vi "Matrix_display_target.vi"() -> ()   [LabVIEW 2013]
uses:
  <vilib>/Platform/TimedLoop/XDataNode/timing_clust.ctl
  <vilib>/Platform/TimedLoop/XDataNode/nitl_modes.ctl
  <vilib>/Platform/TimedLoop/XDataNode/wakeup.ctl
  <vilib>/rvi/Emulation/niFpgaSctlEmulationGetInTimedLoop.vi
  <vilib>/rvi/Emulation/niFpgaProcessEmulError.vi
  <vilib>/rvi/Emulation/niFpgaEmulationReportErrorSimple.vi
  <vilib>/rvi/Emulation/niFpgaGetClockAttributes.vi
  <vilib>/rvi/Emulation/niFpgaCriticalErrorInLSC.vi
  <vilib>/rvi/eio/common/nirviEmuTemplateMethod_errors.vi
  <vilib>/rvi/interface/RandomDataEmulation/nirviRandomDataFPGAFIFO.vi
  <vilib>/rvi/interface/RandomDataEmulation/niFpgaRandomDataHandleErrors.vi
  <vilib>/Platform/TimedLoop/XDataNode/XDataNode.xnode
  <vilib>/eio/EIONode/EIONode.xnode
  <vilib>/rvi/DataTransferAndStorage/Container/XNode/niFpgaContainer.xnode
  <vilib>/rvi/interface/RandomDataEmulation/nirviRandomDataFpgaReadWriteTemplate.vi
  <vilib>/Platform/TimedLoop/XDataNode/XDNodeRunTimeDep.lvlib
panel:
  out "String_counter":i16
  in  "String_number":i16
  in  "I2C_Write":bool
  in  "Read2":u8 format="%x"
  in  "Read1":u8 format="%x"
  in  "Device_Read":u8=187 format="%x"
  in  "Reg":u8=9 format="%x"
  in  "Device_Write":u8=186 format="%x"
  in  "89":i16=89
  in  "100_Sclk_divider":i32=25
  out "Sclk":bool
  in  "75_Stop":i16=75
  in  "53":i16=53
  in  "35":i16=35
  in  "17":i16=17
  in  "71":i16=71
  in  "54":i16=54
  in  "36":i16=36
  in  "18":i16=18
  in  "72":i16=72
  in  "50_Rise/Fall divider":i32=50
  in  "0_WE divider":i32
  in  "DataUp":u64
  in  "DataLow":u64
  out "ACK":bool[](array[boolean])
  out "Data_Array":bool[](array[boolean])
  in  "I2C_Request":bool
  in  "FALSE_LV":bool
  in  "FALSE_PIXCLK":bool
  in  "TRUE_FV":bool
  in  "Линия_ прочтена":bool
  in  "Остановите":bool
  out "Линия_готова_на_все":bool
  in  "Читай_Линию":bool
  in  "1_EXTCLK_divider":i16=2
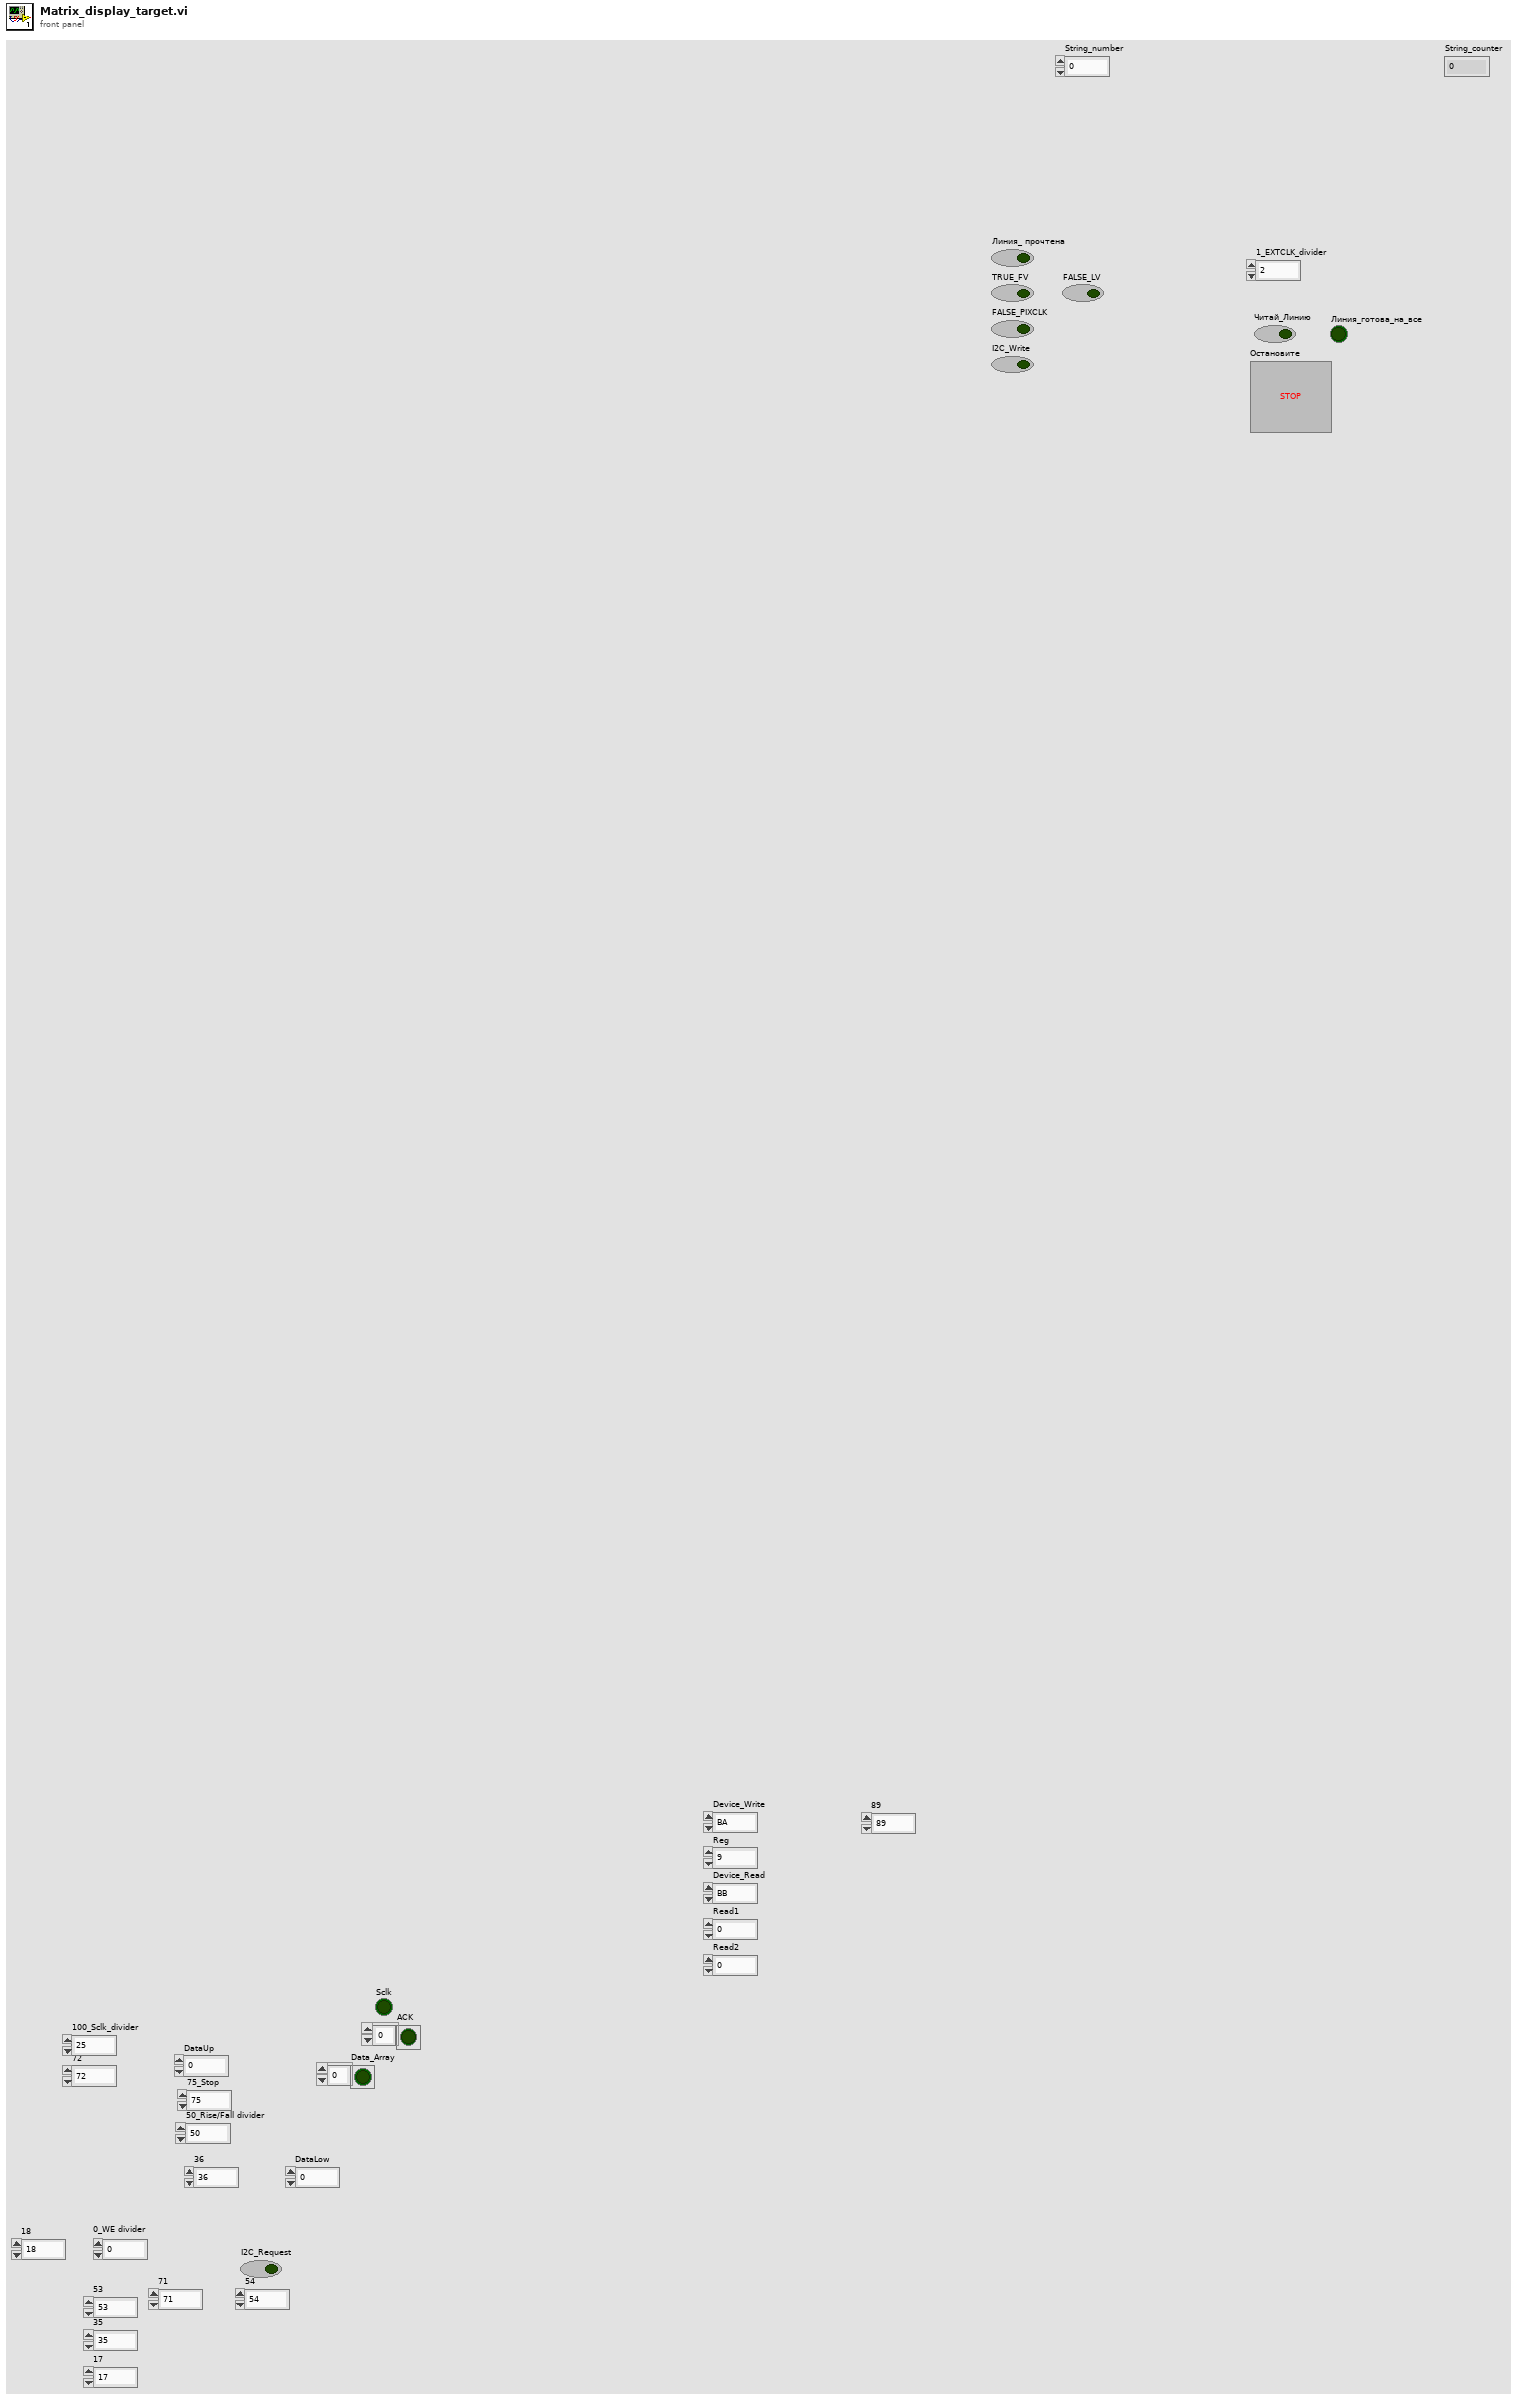
[diagram p1: front panel]
types:
  T1 = typedef "XDNodeRunTimeDep.lvlib/timing_clust.ctl" = cluster{"Expected End [f-1]":u64, "Actual End [f-1]":u64, "Finished Late? [f-1]":bool, "Expected End [i-1]":u64, "Actual End [i-1]":u64, "Finished Late? [i-1]":bool, "Expected Start [i]":u64, "Actual Start [i]":u64, "Expected Start [f]":u64, "Actual Start [f]":u64, "Source Name":string, "Structure Name":string, "Period":i64, "Deadline":i64, "Offset":i64, "Start":i64, "Priority":i32, "Timeout":i32, "Mode":T2, "Wakeup Reason":T3, "Error":errorcluster, "Source Type":string, "Secondary Source Type":string, "Global End Time":u64, "Global Start Time":u64, "Frame Duration":u64, "Iteration Duration":u64, "Assigned CPU":i32, "I/O Scan Engine Mode":u32}
  T2 = typedef "XDNodeRunTimeDep.lvlib/nitl_modes.ctl" = enum32{"No Change", "Process missed periods, maintain original phase", "Discard missed periods, maintain original phase", "Process missed periods, ignore original phase", "Discard missed periods, ignore original phase"}
  T3 = typedef "XDNodeRunTimeDep.lvlib/wakeup.ctl" = enum32{"Normal", "Aborted", "Asynchronous wakeup", "Timing source error", "Timed loop error", "Timeout"}
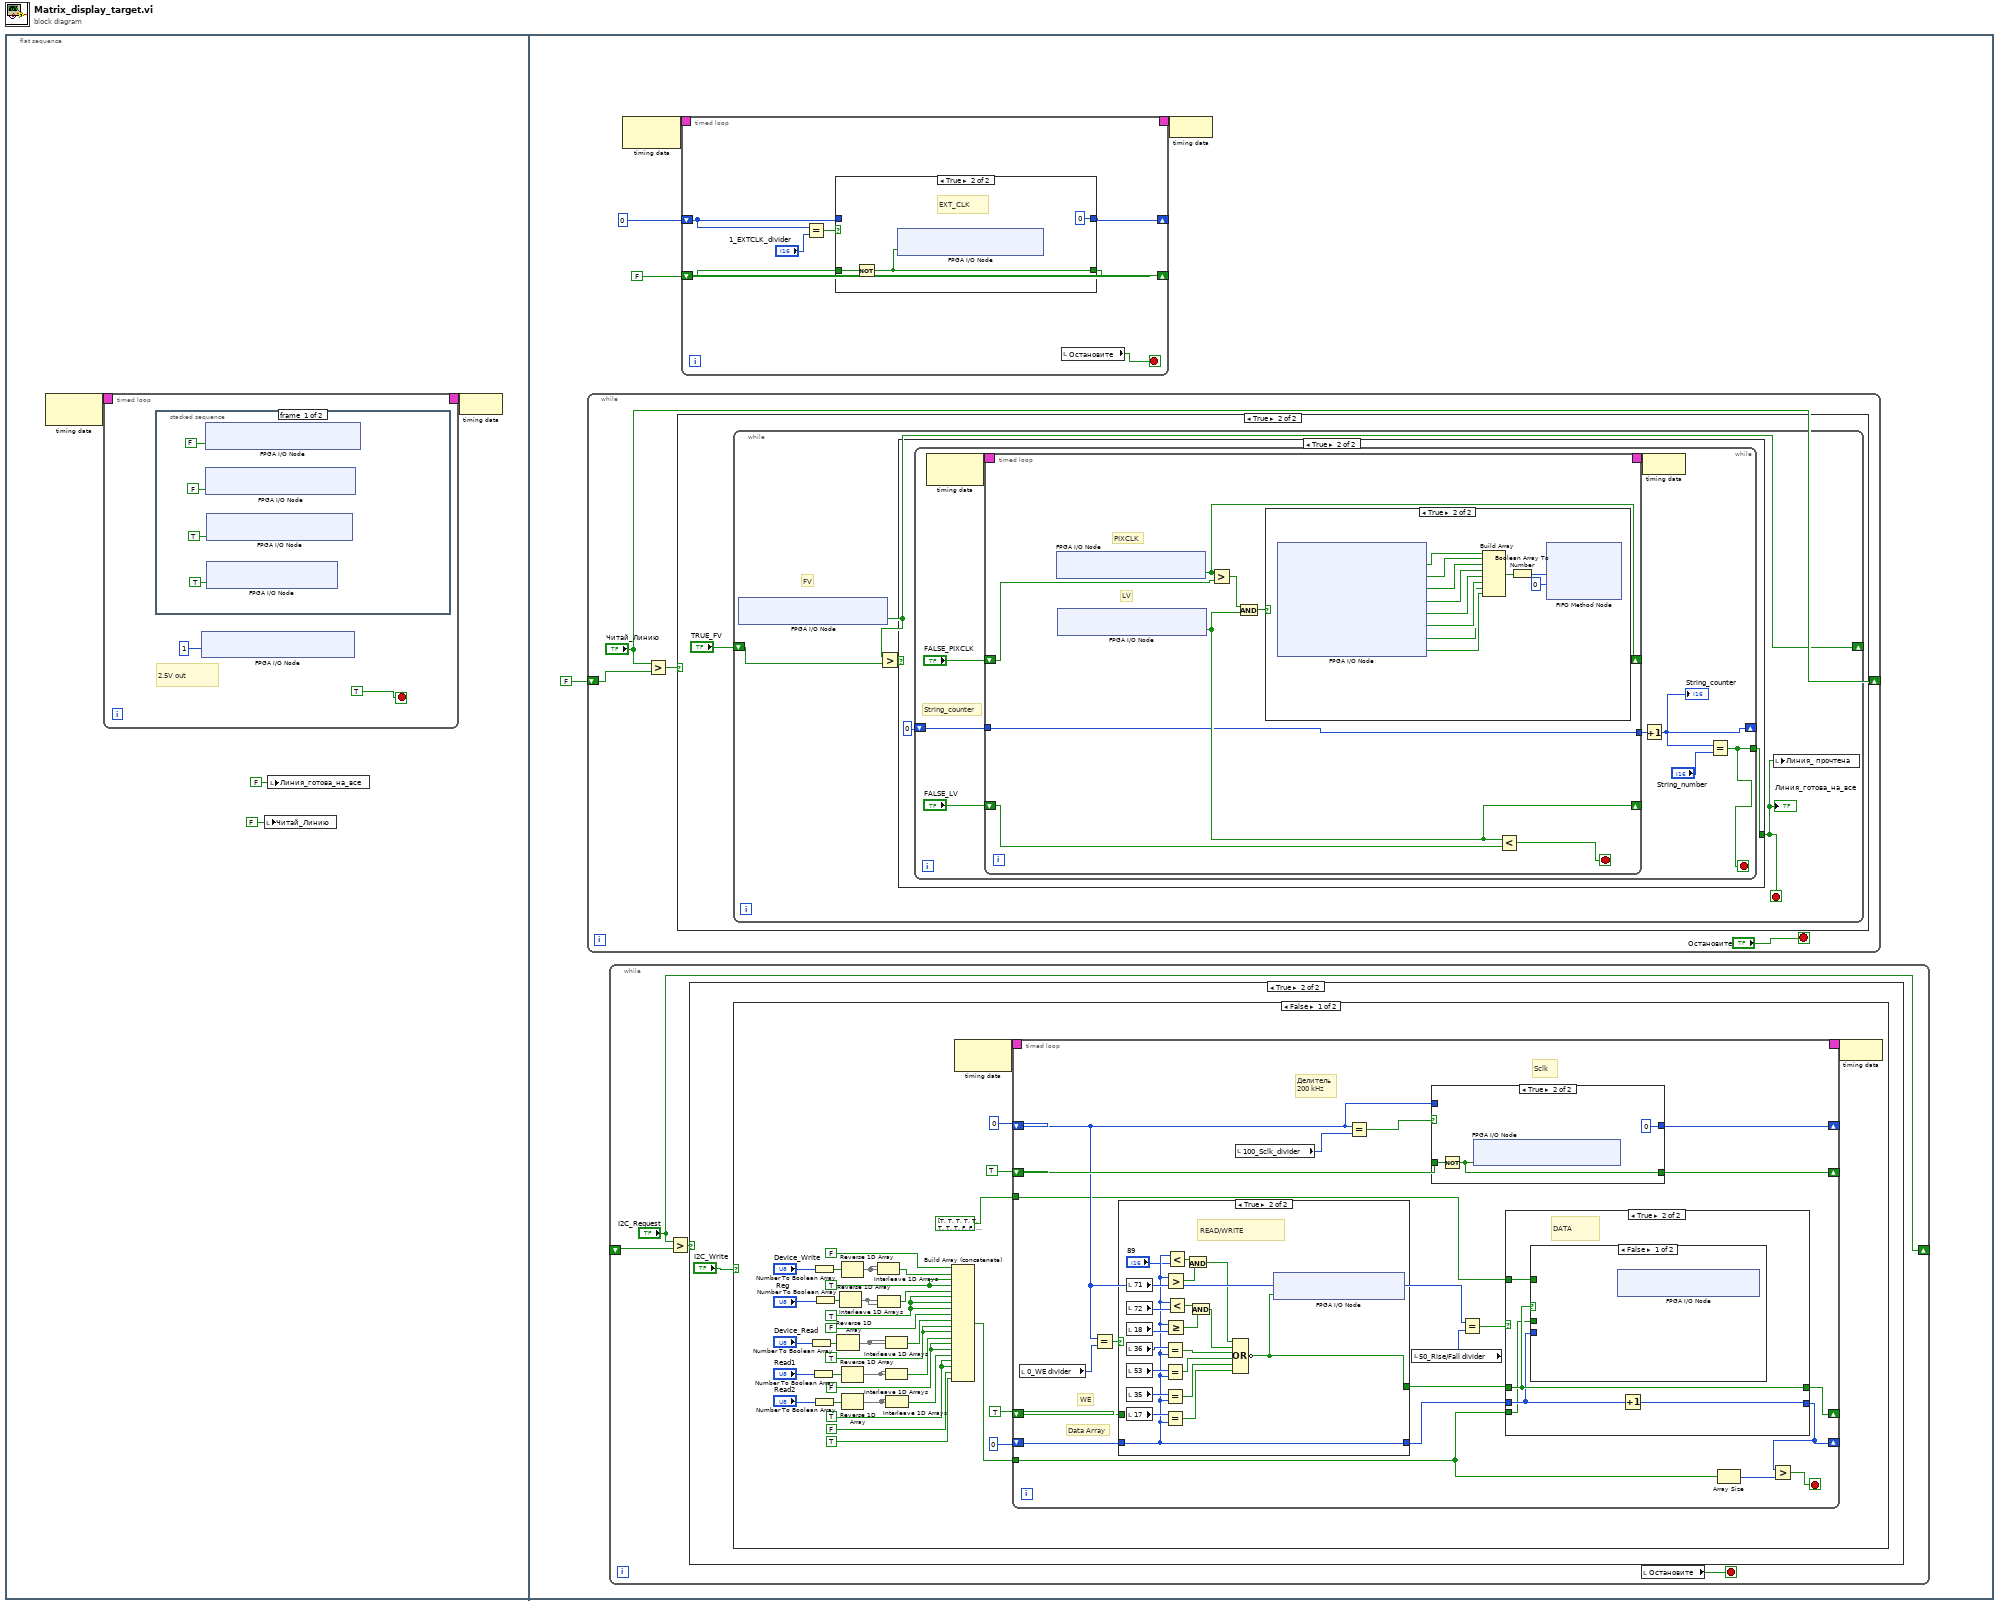
[diagram p0: block diagram]
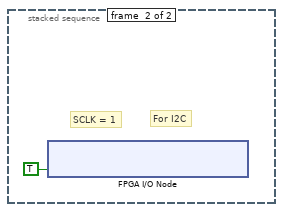
[diagram p2: hidden frame]
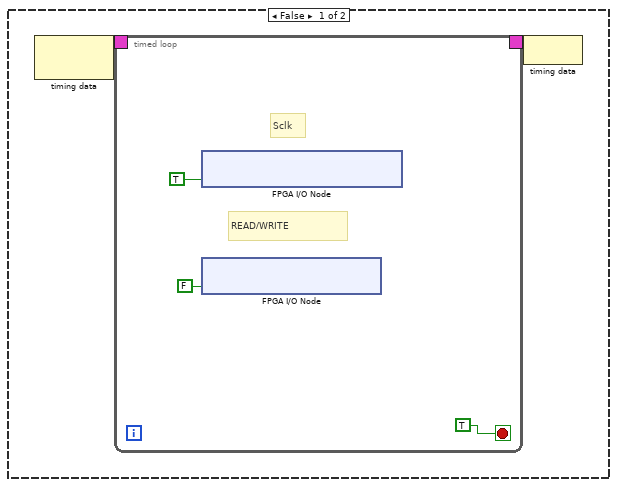
[diagram p3: hidden frame]
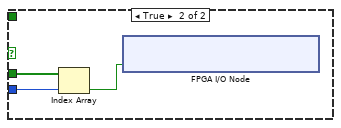
[diagram p6: hidden frame]
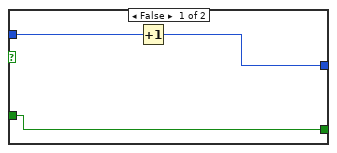
[diagram p7: hidden frame]
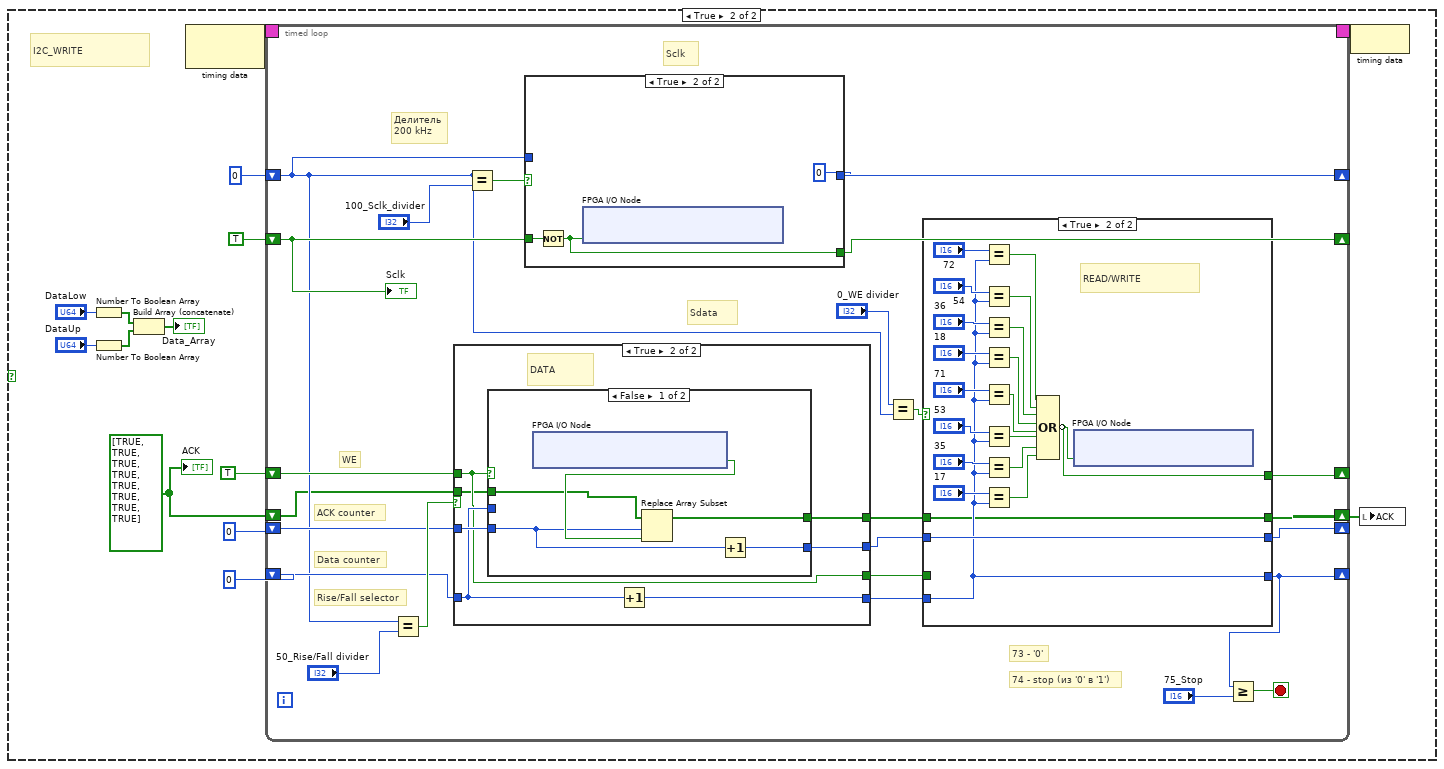
[diagram p8: hidden frame]
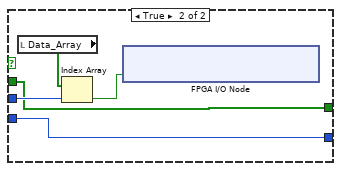
[diagram p11: hidden frame]
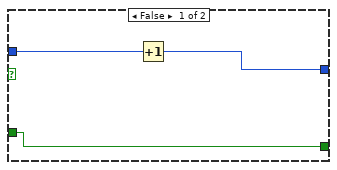
[diagram p12: hidden frame]
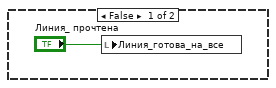
[diagram p13: hidden frame]
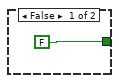
[diagram p14: hidden frame]
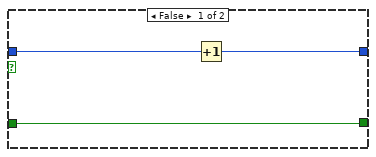
[diagram p16: hidden frame]
diagram:
  n1 = flat-sequence {
    frame #0 {
      n2 = node-c288() -> (w2:T1)  [unwired: 1 in]
      n3 = timed-loop {
        timing: w2 -> [_]
        timing-out: [_] -> w1
        stop <- TRUE stop-if-true
        # "2.5V out"
        n4 = stacked-sequence {
          frame #0 {
            n5 = xnode "FPGA I/O Node"("IO Module\\DDCA_DIO16-23_WE"=FALSE ("IO Module\\DDCA_DIO16-23_WE")) -> ()  [unwired: 1 in, 1 out]
            n6 = xnode "FPGA I/O Node"("IO Module\\DDCA_DIO8-15_WE"=FALSE ("IO Module\\DDCA_DIO8-15_WE")) -> ()  [unwired: 1 in, 1 out]
            n7 = xnode "FPGA I/O Node"("IO Module\\DDCA_DIO0-7_WE"=TRUE ("IO Module\\DDCA_DIO0-7_WE")) -> ()  [unwired: 1 in, 1 out]
            n8 = xnode "FPGA I/O Node"("IO Module\\DDCA_PFI_WE"=TRUE ("IO Module\\DDCA_DIO0-7_WE")) -> ()  [unwired: 1 in, 1 out]
          }
          frame #1 {
            # "For I2C"
            # "SCLK = 1"
            n9 = xnode "FPGA I/O Node"("IO Module\\DDCA_DIO6_Write"=TRUE ("IO Module\\DDCA_DIO6_Write")) -> ()  [unwired: 1 in, 1 out]
          }
        }
        n10 = xnode "FPGA I/O Node"("IO Module\\Local_Supply_Select"=u8 1 ("IO Module\\Local_Supply_Select")) -> ()  [unwired: 1 in, 1 out]
      }
      n11 = local write "Читай_Линию"(FALSE ("Читай_Линию")) -> ()
      n12 = local write "Линия_готова_на_все"(FALSE ("Линия_готова_на_все")) -> ()
      n13 = node-c288(w1) -> ()
    }
    frame #1 {
      n14 = while {
        shift-right: ["Читай_Линию"] -> _
        shift-left: FALSE -> [w229]
        stop <- "Остановите" stop-if-true
        n15 = Greater?(x="Читай_Линию", y=w229) -> (0:w230:bool)
        n16 = case shown="True" w230 {
          frame False {
            n17 = local write "Линия_готова_на_все"("Линия_ прочтена") -> ()
          }
          frame True {
            n18 = while {
              shift-right: [w234] -> _
              shift-left: "TRUE_FV" -> [w235]
              stop <- w233 stop-if-true
              # "FV"
              n19 = xnode "FPGA I/O Node"() -> ("IO Module\\DDCA_DIO23_Read"=w234:bool)  [unwired: 1 in, 1 out]
              n20 = Greater?(x=w234, y=w235) -> (0:w236:bool)
              n21 = case shown="True" w236 {
                tunnel: [FALSE w239] -> w233
                frame False {
                }
                frame True {
                  n22 = while {
                    tunnel: [w240] -> w239
                    shift-right: [w241] -> _
                    shift-left: i16 0 -> [w243]
                    stop <- w240 stop-if-true
                    # "String_counter"
                    n23 = node-c288() -> (w248:T1)  [unwired: 1 in]
                    n24 = timed-loop {
                      timing: w248 -> [_]
                      timing-out: [_] -> w247
                      shift-right: [w254] -> _
                      shift-left: "FALSE_LV" -> [w255]
                      shift-right: [w250] -> _
                      shift-left: "FALSE_PIXCLK" -> [w251]
                      tunnel: w243 -> [w249]
                      tunnel: [w249] -> w242
                      stop <- w253 stop-if-true
                      # "LV"
                      # "PIXCLK"
                      n25 = xnode "FPGA I/O Node"() -> ("IO Module\\DDCA_DIO17_Read"=w250:bool)  [unwired: 1 in, 1 out]
                      n26 = xnode "FPGA I/O Node"() -> ("IO Module\\DDCA_DIO22_Read"=w254:bool)  [unwired: 1 in, 1 out]
                      n27 = Greater?(x=w250, y=w251) -> (0:w252:bool)
                      n28 = Compound Arithmetic op=AND(w252, w254) -> (w256:bool)
                      n29 = case shown="True" w256 {
                        frame False {
                        }
                        frame True {
                          n30 = xnode "FPGA I/O Node"() -> ("IO Module\\DDCA_DIO8_Read"=w265:bool, "IO Module\\DDCA_DIO9_Read"=w264:bool, "IO Module\\DDCA_DIO10_Read"=w263:bool, "IO Module\\DDCA_DIO11_Read"=w262:bool, "IO Module\\DDCA_DIO12_Read"=w261:bool, "IO Module\\DDCA_DIO13_Read"=w260:bool, "IO Module\\DDCA_DIO14_Read"=w259:bool, "IO Module\\DDCA_DIO15_Read"=w258:bool)  [unwired: 8 in, 8 out]
                          n31 = Build Array(w265, w264, w263, w262, w261, w260, w259, w258) -> (w257:bool[])
                          n32 = Boolean Array To Number(Boolean array=w257) -> (number=w266:u8)
                          n33 = xnode ("FIFO Method Node")("Element"=w266, "Timeout"=0) -> ()  [unwired: 1 in, 2 out]
                        }
                      }
                      n34 = Less?(x=w254, y=w255) -> (x < y?=w253:bool)
                    }
                    n35 = node-c288(w247) -> ()
                    n36 = Increment(x=w242) -> (x+1=w241:i16)
                    "String_counter" <- w241
                    n37 = Equal?(x=w241, y="String_number") -> (x = y?=w240:bool)
                  }
                }
              }
              "Линия_готова_на_все" <- w233
              n38 = local write "Линия_ прочтена"(w233) -> ()
            }
          }
        }
      }
      n39 = while {
        shift-right: ["I2C_Request"] -> _
        shift-left: _ -> [w24]
        stop <- w22 stop-if-true
        n40 = Greater?(x="I2C_Request", y=w24) -> (0:w23:bool)
        n41 = case shown="True" w23 {
          frame False {
            n42 = node-c288() -> (w26:T1)  [unwired: 1 in]
            n43 = timed-loop {
              timing: w26 -> [_]
              timing-out: [_] -> w25
              stop <- TRUE stop-if-true
              # "READ/WRITE"
              # "Sclk"
              n44 = xnode "FPGA I/O Node"("IO Module\\DDCA_DIO6_Write"=TRUE) -> ()  [unwired: 1 in, 1 out]
              n45 = xnode "FPGA I/O Node"("IO Module\\DDCA_PFI_WE"=FALSE ("IO Module\\DDCA_PFI_WE")) -> ()  [unwired: 1 in, 1 out]
            }
            n46 = node-c288(w25) -> ()
          }
          frame True {
            n47 = case shown="False" "I2C_Write" {
              frame False {
                w45 = TRUE
                w47 = FALSE
                w51 = TRUE
                w54 = TRUE
                w57 = TRUE
                n48 = Number To Boolean Array(number="Device_Read") -> (Boolean array=w62:bool[])
                n49 = Number To Boolean Array(number="Read1") -> (Boolean array=w42:bool[])
                n50 = Number To Boolean Array(number="Device_Write") -> (Boolean array=w60:bool[])
                n51 = Number To Boolean Array(number="Read2") -> (Boolean array=w41:bool[])
                n52 = Number To Boolean Array(number="Reg") -> (Boolean array=w61:bool[])
                n53 = Reverse 1D Array(array=w62) -> (reversed array=w38:bool[])
                n54 = Reverse 1D Array(array=w61) -> (reversed array=w39:bool[])
                n55 = Reverse 1D Array(array=w60) -> (reversed array=w40:bool[])
                n56 = Reverse 1D Array(array=w42) -> (reversed array=w37:bool[])
                n57 = Reverse 1D Array(array=w41) -> (reversed array=w36:bool[])
                n58 = Interleave 1D Arrays(w40, w40) -> (w58:bool[])
                n59 = Interleave 1D Arrays(w39, w39) -> (w56:bool[])
                n60 = Interleave 1D Arrays(w38, w38) -> (w52:bool[])
                n61 = Interleave 1D Arrays(w37, w37) -> (w48:bool[])
                n62 = Interleave 1D Arrays(w36, w36) -> (w46:bool[])
                n63 = Build Array (concatenate)(FALSE, w58, w57, w57, w56, w54, w54, w54, FALSE, w52, w51, w51, w48, w47, w47, w46, w45, w45, FALSE, TRUE) -> (w55:bool[])
                n64 = node-c288() -> (w71:T1)  [unwired: 1 in]
                n65 = timed-loop {
                  timing: w71 -> [_]
                  timing-out: [_] -> w70
                  shift-right: [w88] -> _
                  shift-left: i16 0 -> [w82]
                  shift-right: [w89] -> _
                  shift-left: TRUE -> [w90]
                  shift-right: [w85] -> _
                  shift-left: TRUE -> [w87]
                  shift-right: [w77] -> _
                  shift-left: i16 0 -> [w81]
                  tunnel: w55 -> [w79]
                  tunnel: bool[] [TRUE, TRUE, TRUE, TRUE, TRUE, TRUE, TRUE, TRUE, FALSE, FALSE, FALSE, FALSE, FALSE, FALSE, FALSE, FALSE] ("ACK") -> [w72]
                  stop <- w78 stop-if-true
                  # "Data Array"
                  # "WE"
                  # "Sclk"
                  # "Делитель\n200 kHz"
                  n66 = local read "0_WE divider"() -> (w73:i32)
                  n67 = Equal?(x=w82, y=w73) -> (x = y?=w84:bool)
                  n68 = case shown="True" w84 {
                    tunnel: [w93 w111] -> w86
                    tunnel: w87 -> [w93 _]
                    tunnel: w81 -> [w92 w95]
                    tunnel: [w92 w95] -> w80
                    frame False {
                    }
                    frame True {
                      # "READ/WRITE"
                      n69 = local read "71"() -> (w96:i16)
                      n70 = local read "72"() -> (w97:i16)
                      n71 = local read "18"() -> (w98:i16)
                      n72 = local read "36"() -> (w99:i16)
                      n73 = local read "53"() -> (w100:i16)
                      n74 = local read "35"() -> (w101:i16)
                      n75 = local read "17"() -> (w102:i16)
                      n76 = Equal?(x=w99, y=w95) -> (x = y?=w109:bool)
                      n77 = Equal?(x=w100, y=w95) -> (x = y?=w110:bool)
                      n78 = Equal?(x=w101, y=w95) -> (x = y?=w112:bool)
                      n79 = Equal?(x=w102, y=w95) -> (x = y?=w113:bool)
                      n80 = Greater?(x=w95, y=w96) -> (0:w105:bool)
                      n81 = Greater Or Equal?(x=w95, y=w98) -> (x >= y?=w107:bool)
                      n82 = Less?(x=w95, y="89") -> (x < y?=w104:bool)
                      n83 = Less?(x=w95, y=w97) -> (x < y?=w108:bool)
                      n84 = And(x=w104, y=w105) -> (x .and. y?=w103:bool)
                      n85 = And(x=w108, y=w107) -> (x .and. y?=w106:bool)
                      n86 = Compound Arithmetic op=OR(w103, w106, w109, w110, w112, w113) -> (invert w111:bool)
                      n87 = xnode "FPGA I/O Node"("IO Module\\DDCA_PFI_WE"=w111) -> ()  [unwired: 1 in, 1 out]
                    }
                  }
                  n88 = local read "100_Sclk_divider"() -> (w75:i32)
                  n89 = Equal?(x=w82, y=w75) -> (x = y?=w91:bool)
                  n90 = local read "50_Rise/Fall divider"() -> (w74:i32)
                  n91 = case shown="True" w91 {
                    tunnel: [w126 0] -> w88
                    tunnel: w90 -> [w125 w128]
                    tunnel: [w125 w127] -> w89
                    tunnel: w82 -> [w124 _]
                    frame False {
                      n92 = Increment(x=w124) -> (x+1=w126:i32)
                    }
                    frame True {
                      n93 = Not(x=w128) -> (.not. x?=w127:bool)
                      n94 = xnode "FPGA I/O Node"("IO Module\\DDCA_DIO6_Write"=w127) -> ()  [unwired: 1 in, 1 out]
                    }
                  }
                  n95 = Equal?(x=w82, y=w74) -> (x = y?=w83:bool)
                  n96 = case shown="True" w83 {
                    tunnel: w86 -> [w115 w120]
                    tunnel: [w115 w120] -> w85
                    tunnel: w80 -> [w114 w119]
                    tunnel: [w114 w118] -> w77
                    tunnel: w79 -> [_ w117]
                    tunnel: w72 -> [_ w116]
                    frame False {
                    }
                    frame True {
                      # "DATA"
                      n97 = case shown="False" w120 {
                        tunnel: w119 -> [_ w123]
                        tunnel: w117 -> [_ w122]
                        tunnel: w116 -> [_ _]
                        frame False {
                          n98 = xnode "FPGA I/O Node"() -> ()  [unwired: 1 in, 2 out]
                        }
                        frame True {
                          n99 = Index Array(array=w122, index=w123) -> (element=w121:bool)
                          n100 = xnode "FPGA I/O Node"("IO Module\\DDCA_PFI2_Write"=w121) -> ()  [unwired: 1 in, 1 out]
                        }
                      }
                      n101 = Increment(x=w119) -> (x+1=w118:i16)
                    }
                  }
                  n102 = Array Size(array=w79) -> (size(s)=w76:i32)
                  n103 = Greater?(x=w77, y=w76) -> (0:w78:bool)
                }
                n104 = node-c288(w70) -> ()
              }
              frame True {
                w134 = bool[] [TRUE, TRUE, TRUE, TRUE, TRUE, TRUE, TRUE, TRUE] ("ACK")
                # "I2C_WRITE"
                n105 = Number To Boolean Array(number="DataLow") -> (Boolean array=w141:bool[])
                n106 = Number To Boolean Array(number="DataUp") -> (Boolean array=w140:bool[])
                n107 = Build Array (concatenate)(w141, w140) -> (→"Data_Array":bool[])
                n108 = node-c288() -> (w147:T1)  [unwired: 1 in]
                n109 = timed-loop {
                  timing: w147 -> [_]
                  timing-out: [_] -> w146
                  shift-right: [w170] -> _
                  shift-left: 0 -> [w159]
                  shift-right: [w169] -> _
                  shift-left: TRUE ("IO Module\\DDCA_DIO0_Write") -> [w166]
                  shift-right: [w156] -> _
                  shift-left: i16 0 -> [w164]
                  shift-right: [w154] -> _
                  shift-left: i16 0 -> [w163]
                  shift-right: [w153] -> _
                  shift-left: TRUE -> [w162]
                  shift-right: [w149] -> w135
                  shift-left: w134 -> [w148]
                  stop <- w151 stop-if-true
                  # "Rise/Fall selector"
                  # "WE"
                  # "Data counter"
                  # "ACK counter"
                  # "74 - stop (из '0' в '1')"
                  # "73 - '0'"
                  # "Sdata"
                  # "Sclk"
                  # "Делитель\n200 kHz"
                  n110 = Equal?(x=w159, y="50_Rise/Fall divider") -> (x = y?=w165:bool)
                  n111 = case shown="True" w165 {
                    tunnel: [w198 w202] -> w157
                    tunnel: w164 -> [w198 w204]
                    tunnel: w163 -> [w199 w206]
                    tunnel: [w199 w205] -> w155
                    tunnel: w162 -> [w197 w203]
                    tunnel: [w197 w203] -> w152
                    tunnel: [w196 w201] -> w150
                    tunnel: w148 -> [w196 w200]
                    frame False {
                    }
                    frame True {
                      # "DATA"
                      n112 = case shown="False" w203 {
                        tunnel: w206 -> [w210 w216]
                        tunnel: [w209 w216] -> w205
                        tunnel: w204 -> [_ w215]
                        tunnel: [w208 w212] -> w201
                        tunnel: w200 -> [w207 w212]
                        frame False {
                          n113 = xnode "FPGA I/O Node"() -> ("IO Module\\DDCA_PFI2_Read"=w211:bool)  [unwired: 1 in, 1 out]
                          n114 = Replace Array Subset(array=w207, new element=w211, index=w210) -> (w208:bool[])
                          n115 = Increment(x=w210) -> (x+1=w209:i16)
                        }
                        frame True {
                          n116 = local read "Data_Array"() -> (w214:bool[])
                          n117 = Index Array(array=w214, index=w215) -> (element=w213:bool)
                          n118 = xnode "FPGA I/O Node"("IO Module\\DDCA_PFI2_Write"=w213) -> ()  [unwired: 1 in, 1 out]
                        }
                      }
                      n119 = Increment(x=w204) -> (x+1=w202:i16)
                    }
                  }
                  n120 = Equal?(x=w159, y="100_Sclk_divider") -> (x = y?=w171:bool)
                  n121 = case shown="True" w171 {
                    tunnel: [w218 0] -> w170
                    tunnel: w159 -> [w219 _]
                    tunnel: w166 -> [w217 w221]
                    tunnel: [w217 w220] -> w169
                    frame False {
                      n122 = Increment(x=w219) -> (x+1=w218:i32)
                    }
                    frame True {
                      n123 = Not(x=w221) -> (.not. x?=w220:bool)
                      n124 = xnode "FPGA I/O Node"("IO Module\\DDCA_DIO6_Write"=w220) -> ()  [unwired: 1 in, 1 out]
                    }
                  }
                  n125 = Equal?(x="0_WE divider", y=w159) -> (x = y?=w158:bool)
                  n126 = case shown="True" w158 {
                    tunnel: w157 -> [w174 w181]
                    tunnel: [w174 w181] -> w156
                    tunnel: [w175 w187] -> w154
                    tunnel: w155 -> [w175 w187]
                    tunnel: [w173 w186] -> w153
                    tunnel: w152 -> [w173 _]
                    tunnel: w150 -> [w172 w176]
                    tunnel: [w172 w176] -> w149
                    frame False {
                    }
                    frame True {
                      # "READ/WRITE"
                      n127 = Equal?(x="72", y=w181) -> (x = y?=w180:bool)
                      n128 = Equal?(x="54", y=w181) -> (x = y?=w177:bool)
                      n129 = Equal?(x="36", y=w181) -> (x = y?=w179:bool)
                      n130 = Equal?(x="18", y=w181) -> (x = y?=w178:bool)
                      n131 = Equal?(x="71", y=w181) -> (x = y?=w188:bool)
                      n132 = Equal?(x="53", y=w181) -> (x = y?=w191:bool)
                      n133 = Equal?(x="35", y=w181) -> (x = y?=w193:bool)
                      n134 = Equal?(x="17", y=w181) -> (x = y?=w195:bool)
                      n135 = Compound Arithmetic op=OR(w180, w177, w179, w178, w188, w191, w193, w195) -> (invert w186:bool)
                      n136 = xnode "FPGA I/O Node"("IO Module\\DDCA_PFI_WE"=w186) -> ()  [unwired: 1 in, 1 out]
                    }
                  }
                  n137 = Greater Or Equal?(x=w156, y="75_Stop") -> (x >= y?=w151:bool)
                  "Sclk" <- w166
                }
                n138 = node-c288(w146) -> ()
                n139 = local write "ACK"(w135) -> ()
                "ACK" <- w134
              }
            }
          }
        }
        n140 = local read "Остановите"() -> (w22:bool)
      }
      n141 = node-c288() -> (w20:T1)  [unwired: 1 in]
      n142 = timed-loop {
        timing: w20 -> [_]
        timing-out: [_] -> w19
        shift-right: [w273] -> _
        shift-left: i16 0 -> [w275]
        shift-right: [w274] -> _
        shift-left: FALSE -> [w276]
        stop <- w272 stop-if-true
        n143 = Equal?(x=w275, y="1_EXTCLK_divider") -> (x = y?=w278:bool)
        n144 = case shown="True" w278 {
          tunnel: w276 -> [w279 w284]
          tunnel: [w279 w283] -> w274
          tunnel: w275 -> [w281 _]
          tunnel: [w280 i16 0] -> w273
          frame False {
            n145 = Increment(x=w281) -> (x+1=w280:i16)
          }
          frame True {
            # "EXT_CLK"
            n146 = Not(x=w284) -> (.not. x?=w283:bool)
            n147 = xnode "FPGA I/O Node"("IO Module\\DDCA_DIO7_Write"=w283) -> ()  [unwired: 1 in, 1 out]
          }
        }
        n148 = local read "Остановите"() -> (w272:bool)
      }
      n149 = node-c288(w19) -> ()
    }
  }
